vi "mergeDeviceScriptLists.vi"(8 "error in (no error)":errorcluster, 10 "device":refnum<class "device.lvclass">, 11 "DeviceArray in":refnum<class "DeviceArray.lvclass">) -> (0 "error out":errorcluster, 3 "DeviceArray out":refnum<class "DeviceArray.lvclass">)   [LabVIEW 2009, in "Tools.lvlib" / "DatabaseHelpers.lvlib" / "DeviceArray.lvclass"]
uses:
  DeviceArray.lvclass
  device/device.lvclass
  Scripting/ScriptingEvent/ScriptEventList/ScriptEventList.lvclass
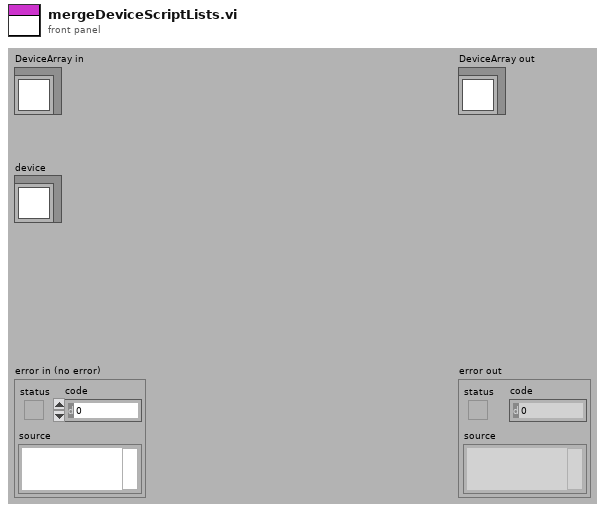
[diagram p1: front panel]
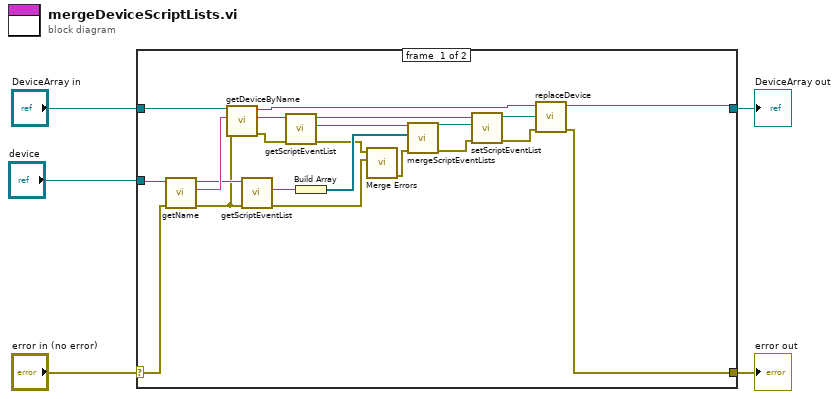
[diagram p0: block diagram]
diagram:
  n1 = case shown="No Error" "error in (no error)" {
    selector: "error in (no error)" -> [w25 w29]
    tunnel: [w7 w29] -> w4
    tunnel: [w6 w28] -> w2
    tunnel: "DeviceArray in" -> [w27 w28]
    tunnel: "device" -> [w26 _]
    frame #0 {
      n2 = call "getName.vi"("error in (no error)"=w25, "device.lvclass in"=w26) -> ("error out"=w22:errorcluster, "name"=w24:string, "device.lvclass out"=w23:refnum<class "device.lvclass">)  [unwired: 7 in]
      n3 = call "getDeviceByName.vi"("error in (no error)"=w22, "deviceName"=w24, "DeviceArray in"=w27) -> ("error out"=w20:errorcluster, "device.lvclass"=w21:refnum<class "device.lvclass">, "DeviceArray out"=w9:refnum<class "DeviceArray.lvclass">)  [unwired: 5 in, 1 out]
      n4 = call "getScriptEventList.vi"("error in (no error)"=w22, "device.lvclass in"=w23) -> ("error out"=w14:errorcluster, "ScriptEventList"=w18:refnum<class "ScriptEventList.lvclass">)  [unwired: 7 in, 1 out]
      n5 = call "getScriptEventList.vi"("error in (no error)"=w20, "device.lvclass in"=w21) -> ("error out"=w15:errorcluster, "ScriptEventList"=w19:refnum<class "ScriptEventList.lvclass">, "device.lvclass out"=w13:refnum<class "device.lvclass">)  [unwired: 7 in]
      n6 = Build Array(w18) -> (w17:refnum<class "ScriptEventList.lvclass">[])
      n7 = call <vilib>:"Merge Errors.vi"("error in 2 (no error)"=w14, "error in 1 (no error)"=w15) -> ("error out"=w16:errorcluster)  [unwired: 5 in]
      n8 = call "mergeScriptEventLists.vi"("error in (no error)"=w16, "Array"=w17, "ScriptEventList in"=w19) -> ("error out"=w11:errorcluster, "ScriptEventList out"=w12:refnum<class "ScriptEventList.lvclass">)  [unwired: 7 in]
      n9 = call "setScriptEventList.vi"("error in (no error)"=w11, "ScriptEventList"=w12, "device.lvclass in"=w13) -> ("error out"=w8:errorcluster, "device.lvclass out"=w10:refnum<class "device.lvclass">)  [unwired: 7 in]
      n10 = call "replaceDevice.vi"("error in (no error)"=w8, "device"=w10, "DeviceArray in"=w9) -> ("error out"=w7:errorcluster, "DeviceArray out"=w6:refnum<class "DeviceArray.lvclass">)  [unwired: 7 in]
    }
    frame #1 {
    }
  }
  "error out" <- w4
  "DeviceArray out" <- w2
